vi "To String.vi"(8 "error in (no error)":errorcluster, 11 "Data Class Array in":refnum<class "Data Class Array.lvclass">) -> (0 "error out":errorcluster, 2 "String":string)   [LabVIEW 2020, in "Data.lvlib" / "Data Class Array.lvclass"]
doc: "Convert 'Generic Data in' to a string."
uses:
  Data Class Array.lvclass
  Data Class Array.lvclass/Data Class Array.ctl
  Data Class/Data Class.lvclass
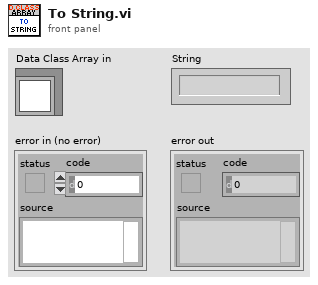
[diagram p1: front panel]
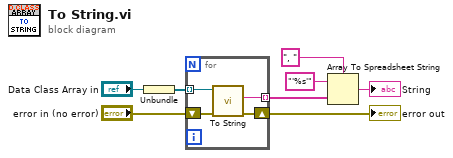
[diagram p0: block diagram]
diagram:
  n1 = Unbundle("Data Class Array in") -> (w4:refnum<class "Data Class.lvclass">[])
  n2 = for {
    tunnel: w4 -> [w12] mode=indexing
    tunnel: [w11] -> w3 mode=indexing
    shift-right: [w9] -> w1
    shift-left: "error in (no error)" -> [w10]
    n3 = call-dynamic "To String.vi"("error in (no error)"=w10, "Data Class in"=w12) -> ("error out"=w9:errorcluster, "String"=w11:string)  [unwired: 8 in]
  }
  "error out" <- w1
  n4 = Array To Spreadsheet String(delimiter (Tab)=", ", array=w3, 3:"'%s'" ("format string")) -> (spreadsheet string=→"String":string)
